vi "SeCrTs-Data Transfer Loop RD.vi"(11 "Data FIFO Ref":T1) -> ()   [LabVIEW 2022 SP3]
uses:
  RT Controls/SeCrTs-Data FIFO.ctl
  RT Controls/SeCrTs-DiplayPC comm ctrl.ctl
  <vilib>/Platform/TimedLoop/XDataNode/timing_clust.ctl
  <vilib>/Platform/TimedLoop/XDataNode/nitl_modes.ctl
  <vilib>/Platform/TimedLoop/XDataNode/wakeup.ctl
  RT Support/SeCrTs-RT_Global_R.vi
  <vilib>/platform/TimedLoop/XDataNode/XDataNode.xnode
  <resource>/objmgr/ni.dex.rc
  <vilib>/Platform/TimedLoop/XDataNode/XDNodeRunTimeDep.lvlib
panel:
  out "length":i32
  out "Available Elements for Writing":i32
  out "Buffer Size":i32
  out "x-y 3":i32
  out "Available Elements for Writing":i32
  out "Buffer Size":i32
  out "x-y 2":i32
  out "x-y":u32
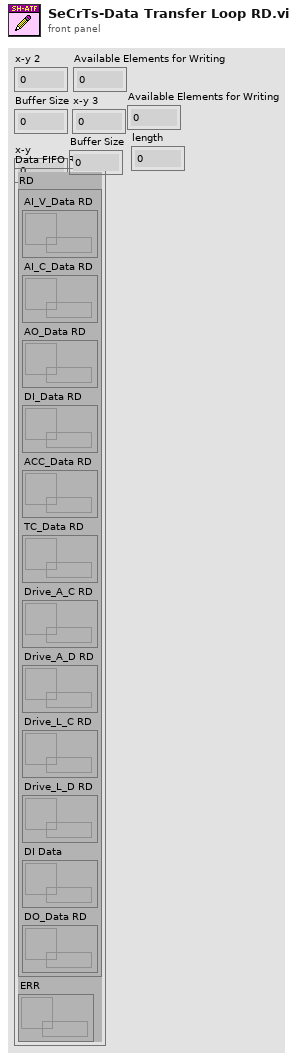
[diagram p1: front panel]
types:
  T1 = typedef "SeCrTs-Data FIFO.ctl" = cluster{"RD":cluster{"AI_V_Data RD":refnum<queue>, "AI_C_Data RD":refnum<queue>, "AO_Data RD":refnum<queue>, "DI_Data RD":refnum<queue>, "ACC_Data RD":refnum<queue>, "TC_Data RD":refnum<queue>, "Drive_A_C RD":refnum<queue>, "Drive_A_D RD":refnum<queue>, "Drive_L_C RD":refnum<queue>, "Drive_L_D RD":refnum<queue>, "DI Data":refnum<queue>, "DO_Data RD":refnum<queue>}, "ERR":refnum<queue>}
  T2 = typedef "SeCrTs-DiplayPC comm ctrl.ctl" = enum16{"Initialize", "Listen for UI Writer", "Send RT Data"}
  T3 = typedef "XDNodeRunTimeDep.lvlib/timing_clust.ctl" = cluster{"Expected End [f-1]":u64, "Actual End [f-1]":u64, "Finished Late? [f-1]":bool, "Expected End [i-1]":u64, "Actual End [i-1]":u64, "Finished Late? [i-1]":bool, "Expected Start [i]":u64, "Actual Start [i]":u64, "Expected Start [f]":u64, "Actual Start [f]":u64, "Source Name":string, "Structure Name":string, "Period":i64, "Deadline":i64, "Offset":i64, "Start":i64, "Priority":i32, "Timeout":i32, "Mode":T4, "Wakeup Reason":T5, "Error":errorcluster, "Source Type":string, "Secondary Source Type":string, "Global End Time":u64, "Global Start Time":u64, "Frame Duration":u64, "Iteration Duration":u64, "Assigned CPU":i32, "I/O Scan Engine Mode":u32}
  T4 = typedef "XDNodeRunTimeDep.lvlib/nitl_modes.ctl" = enum32{"No Change", "Process missed periods, maintain original phase", "Discard missed periods, maintain original phase", "Process missed periods, ignore original phase", "Discard missed periods, ignore original phase"}
  T5 = typedef "XDNodeRunTimeDep.lvlib/wakeup.ctl" = enum32{"Normal", "Aborted", "Asynchronous wakeup", "Timing source error", "Timed loop error", "Timeout"}
  T6 = cluster{"Start DAQ":bool, "Stop DAQ":bool, "RT Stop":bool, "RT Exit":bool, "Start Seq":bool}
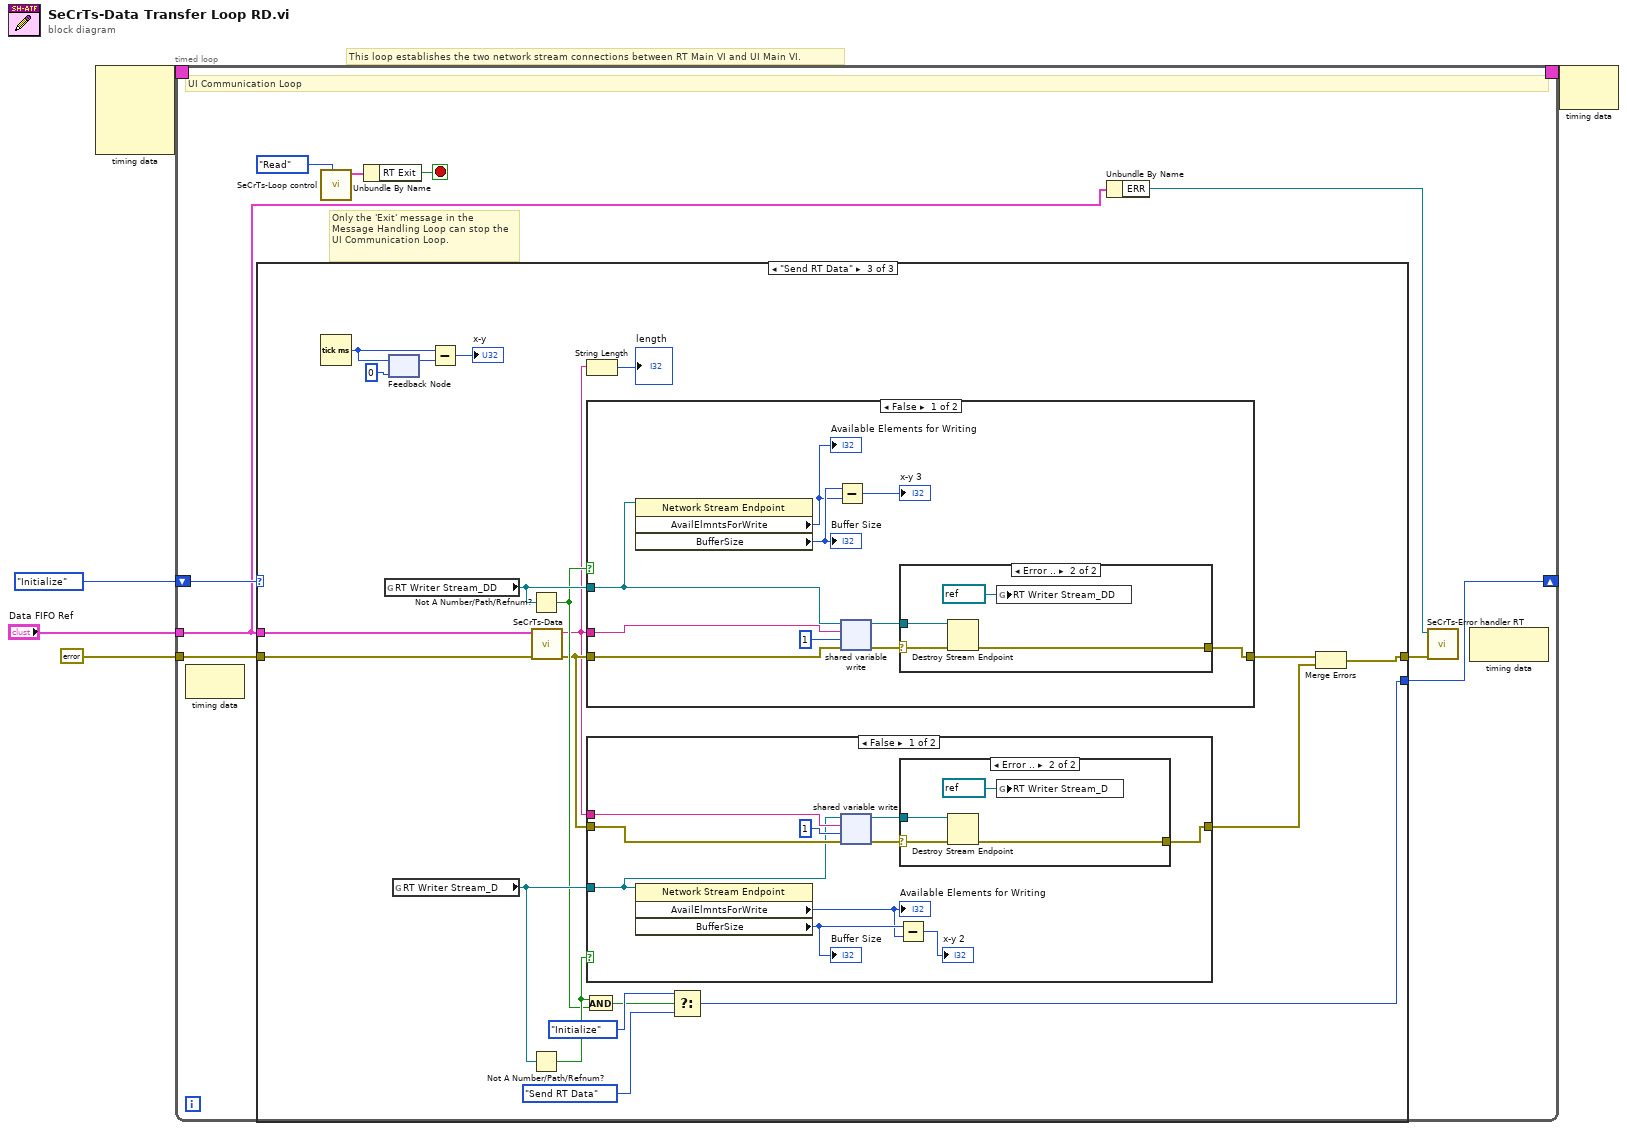
[diagram p0: block diagram]
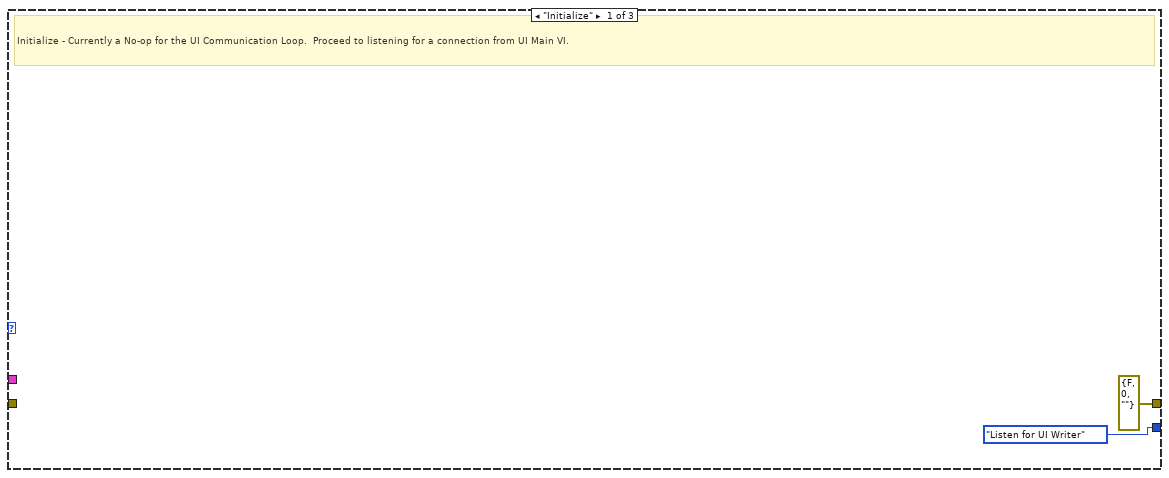
[diagram p2: hidden frame]
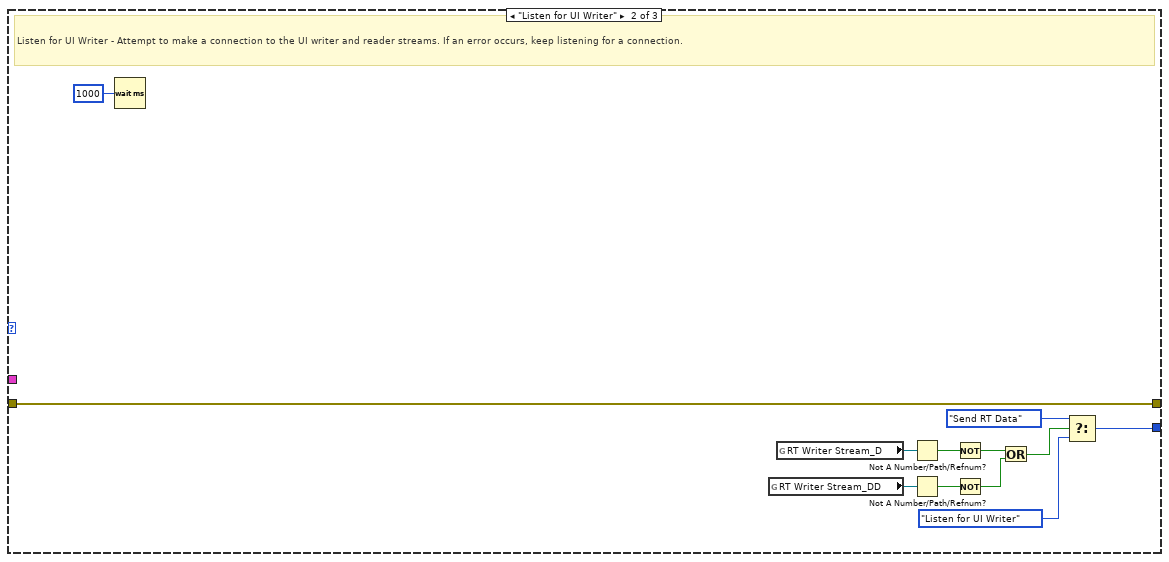
[diagram p3: hidden frame]
diagram:
  # "This loop establishes the two network stream connections between RT Main VI and UI Main VI."
  n1 = node-c288() -> (w2:T3)  [unwired: 4 in]
  n2 = timed-loop {
    shift-right: [w14] -> _
    shift-left: SeCrTs-DiplayPC_comm_ctrl."Initialize" -> [w13]
    tunnel: "Data FIFO Ref" -> [w7]
    tunnel: errorcluster {"status"=FALSE, "code"=0, "source"=""} ("error in (no error)") -> [w8]
    timing: w2 -> [_]
    timing-out: [_] -> w1
    stop <- w10 stop-if-true
    # "Only the 'Exit' message in the  Message Handling Loop can stop the UI Communication Loop."
    # "UI Communication Loop"
    n3 = node-c288() -> ()  [unwired: 1 in, 1 out]
    n4 = case shown="\"Send RT Data\"" w13 {
      tunnel: [errorcluster {"status"=FALSE, "code"=0, "source"=""} ("error IO") w19 w35] -> w9
      tunnel: [SeCrTs-DiplayPC_comm_ctrl."Listen for UI Writer" w24 w46] -> w14
      tunnel: w7 -> [_ _ w37]
      tunnel: w8 -> [_ w19 w38]
      frame "Initialize" {
        # "Initialize - Currently a No-op for the UI Communication Loop.  Proceed to listening for a connection from UI Main VI."
      }
      frame "Listen for UI Writer" {
        # "Listen for UI Writer - Attempt to make a connection to the UI writer and reader streams. If an error occurs, keep listening for a connection."
        n5 = Wait (ms)(milliseconds to wait=u32 1000) -> ()  [unwired: 1 out]
        n6 = global read "SeCrTs-RT_Global_R.vi" "RT Writer Stream_DD"() -> (w29:refnum<k21>)
        n7 = global read "SeCrTs-RT_Global_R.vi" "RT Writer Stream_D"() -> (w30:refnum<k21>)
        n8 = Not A Number/Path/Refnum?(number/path/refnum=w30) -> (NaN/Path/Refnum?=w28:bool)
        n9 = Not A Number/Path/Refnum?(number/path/refnum=w29) -> (NaN/Path/Refnum?=w27:bool)
        n10 = Not(x=w28) -> (.not. x?=w26:bool)
        n11 = Not(x=w27) -> (.not. x?=w25:bool)
        n12 = Or(x=w26, y=w25) -> (x .or. y?=w21:bool)
        n13 = Select(t=SeCrTs-DiplayPC_comm_ctrl."Send RT Data", s=w21, f=SeCrTs-DiplayPC_comm_ctrl."Listen for UI Writer") -> (s? t:f=w24:T2)
      }
      frame "Send RT Data" {
        n14 = Tick Count (ms)() -> (millisecond timer value=w43:u32)
        n15 = global read "SeCrTs-RT_Global_R.vi" "RT Writer Stream_DD"() -> (w44:refnum<k21>)
        n16 = feedback-in #1(w43) -> ()
        n17 = feedback #1(u32 0 ("millisecond timer value")) -> (w42:u32)
        n18 = global read "SeCrTs-RT_Global_R.vi" "RT Writer Stream_D"() -> (w50:refnum<k21>)
        n19 = Subtract(x=w43, y=w42) -> (x-y=→"x-y":u32)
        n20 = Not A Number/Path/Refnum?(number/path/refnum=w44) -> (NaN/Path/Refnum?=w39:bool)
        n21 = Not A Number/Path/Refnum?(number/path/refnum=w50) -> (NaN/Path/Refnum?=w45:bool)
        n22 = call "SeCrTs-Data.vi"("error in (no error)"=w38, "Data FIFO Ref"=w37) -> ("error out"=w33:errorcluster, "data"=w32:string)  [unwired: 8 in]
        n23 = And(x=w45, y=w39) -> (x .and. y?=w47:bool)
        n24 = String Length(string=w32) -> (length=→"length":i32)
        n25 = case shown="False" w39 {
          tunnel: w44 -> [w51 _]
          tunnel: w33 -> [w58 w66]
          tunnel: [w57 w66] -> w40
          tunnel: w32 -> [w56 _]
          frame False {
            n26 = property class="Network Stream Endpoint"(reference=w51) -> ("AvailElmntsForWrite"=w52:i32, "BufferSize"=w53:i32)  [unwired: 1 in, 2 out]
            "Buffer Size" <- w53
            "Available Elements for Writing" <- w52
            n27 = Subtract(x=w53, y=w52) -> (x-y=→"x-y 3":i32)
            n28 = shared-variable-write(w51, w58, w56, 1 ("timeout ms (-1)")) -> (w59:refnum<k21>, w60:errorcluster)  [unwired: 1 out]
            n29 = case shown="Error .." w60 {
              selector: w60 -> [w61 w64]
              tunnel: w59 -> [_ w65]
              tunnel: [w61 w62] -> w57
              frame No Error {
              }
              frame Error {
                n30 = Destroy Stream Endpoint(8:w64, 11:w65) -> (0:w62:errorcluster)
                n31 = global write "SeCrTs-RT_Global_R.vi" "RT Writer Stream_DD"(refnum<k21> refnum ("RT Writer Stream_DD")) -> ()
              }
            }
          }
          frame True {
          }
        }
        n32 = case shown="False" w45 {
          tunnel: w50 -> [w70 _]
          tunnel: w33 -> [w73 w82]
          tunnel: [w74 w82] -> w34
          tunnel: w32 -> [w72 _]
          frame False {
            n33 = property class="Network Stream Endpoint"(reference=w70) -> ("AvailElmntsForWrite"=w67:i32, "BufferSize"=w68:i32)  [unwired: 1 in, 2 out]
            "Buffer Size" <- w68
            "Available Elements for Writing" <- w67
            n34 = shared-variable-write(w70, w73, w72, 1 ("timeout ms (-1)")) -> (w75:refnum<k21>, w76:errorcluster)  [unwired: 1 out]
            n35 = Subtract(x=w68, y=w67) -> (x-y=→"x-y 2":i32)
            n36 = case shown="Error .." w76 {
              selector: w76 -> [w77 w80]
              tunnel: w75 -> [_ w81]
              tunnel: [w77 w78] -> w74
              frame No Error {
              }
              frame Error {
                n37 = Destroy Stream Endpoint(8:w80, 11:w81) -> (0:w78:errorcluster)
                n38 = global write "SeCrTs-RT_Global_R.vi" "RT Writer Stream_D"(refnum<k21> refnum ("RT Writer Stream_DD")) -> ()
              }
            }
          }
          frame True {
          }
        }
        n39 = Select(t=SeCrTs-DiplayPC_comm_ctrl."Initialize", s=w47, f=SeCrTs-DiplayPC_comm_ctrl."Send RT Data") -> (s? t:f=w46:T2)
        n40 = Merge Errors(w40, w34) -> (w35:errorcluster)
      }
    }
    n41 = call "SeCrTs-Loop control.vi"("Action"=enum16{"Init", "Write", "Read"}."Read") -> ("Loop Control out"=w12:T6)  [unwired: 9 in, 1 out]
    n42 = Unbundle By Name(w12) -> ("RT Exit"=w10:bool)
    n43 = Unbundle By Name(w7) -> ("ERR"=w6:refnum<queue>)
    n44 = call "SeCrTs-Error handler RT.vi"("error in"=w9, "Message Queue"=w6) -> ()  [unwired: 8 in, 2 out]
    n45 = node-c288() -> ()  [unwired: 1 in, 1 out]
  }
  n46 = node-c288(w1) -> ()  [unwired: 1 out]
